vi "add_light-dark_j-t_measurements_to_queue.vi"(10 "Scan settings array":T3[](array[typedef]) {"J-t Illumination conditions" items=["Light only", "Dark only", "Light then dark", "Dark then light"]; "No. of scan rate steps" min=1.0 step=1.0; "Illumination conditions" items=["Light only", "Dark only", "Light then dark", "Dark then light", "Light then dark then light", "Dark then light then dark"]; "Only repeat for best pixel" items=["only for best pixel", "for best 2 pixels", "for best 3 pixels", "for best 4 pixels", "for best 5 pixels", "for best 6 pixels", "for best 7 pixels", "for all pixels"]; "No. of repeat scans" min=1.0 step=1.0; "Max power best pixel only" items=["only the best pixel", "the best 2 pixels", "the best 3 pixels", "the best 4 pixels", "the best 5 pixels", "the best 6 pixels", "the best 7 pixels", "all pixels"]; "J-t best pixel only" items=["only the best pixel", "the best 2 pixels", "the best 3 pixels", "the best 4 pixels", "the best 5 pixels", "the best 6 pixels", "the best 7 pixels", "all pixels"]; "Integration time" items=["Fast", "Normal", "High Accuracy"]; "Stabilisation mode" items=["V", "I"]; "Measurement delay (ms)" min=10.0}, 11 "Cell settings cluster":T2) -> (3 "Light/dark array":T1(array[cluster]))   [LabVIEW 2016]
uses:
  TypeDefs/scan_settings.ctl
  TypeDefs/Settings Boolean.ctl
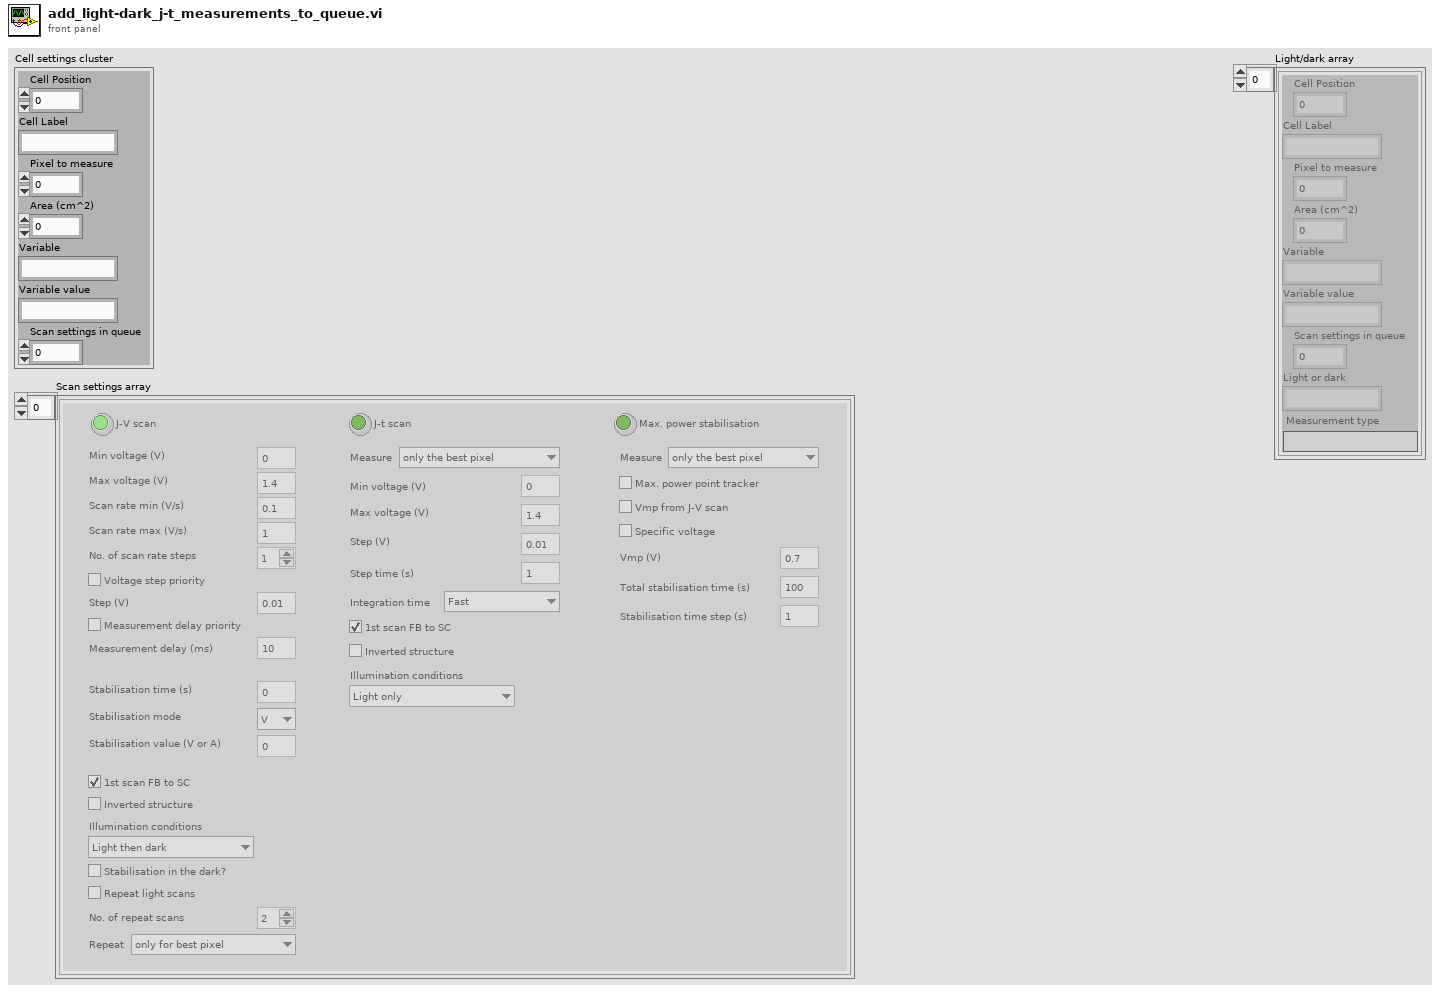
[diagram p1: front panel]
types:
  T1 = cluster{"Cell Position":i32, "Cell Label":string, "Pixel to measure":u16, "Area (cm^2)":dbl, "Variable":string, "Variable value":string, "Scan settings in queue":u16, "Light or dark":string, "Measurement type":string}[]
  T2 = cluster{"Cell Position":i32, "Cell Label":string, "Pixel to measure":u16, "Area (cm^2)":dbl, "Variable":string, "Variable value":string, "Scan settings in queue":u16}
  T3 = typedef "scan_settings.ctl" = cluster{"J-V scan":T4, "J-t scan":bool, "Min voltage (V)":dbl, "Max voltage (V)":dbl, "Step (V)":dbl, "Measurement delay (ms)":dbl, "1st scan FB-SC":bool, "Inverted structure":bool, "Stabilisation time (s)":dbl, "Stabilisation mode":u16, "Stabilisation value (V or A) ":dbl, "Step time (s)":dbl, "Integration time":u16, "Repeat light scans":bool, "Stabilisation in the dark?":bool, "J-t Min (V)":dbl, "J-t Max (V)":dbl, "J-t Step (V)":dbl, "Max. power stabilisation":bool, "J-t 1st scan FB-SC":bool, "J-t Inverted structure":bool, "Max power tracking":bool, "Vmp (V)":dbl, "Total stabilisation time (s)":dbl, "J-t best pixel only":u16, "Max power best pixel only":u16, "Vmp from J-V scan":bool, "No. of repeat scans":dbl, "Only repeat for best pixel":u16, "Stabilisation time step (s)":dbl, "Illumination conditions":u16, "Scan rate min (V/s)":dbl, "Scan rate max (V/s)":dbl, "No. of scan rate steps":dbl, "Scan rate voltage step priority":bool, "Scan rate measurement delay priority":bool, "J-t Illumination conditions":u16, "Max P stab. Specific voltage":bool}
  T4 = typedef "Settings Boolean.ctl" = bool
  T5 = cluster{"Cell Position":i32, "Cell Label":string, "Pixel to measure":u16, "Area (cm^2)":dbl, "Variable":string, "Variable value":string, "Scan settings in queue":u16, "Light or dark":string, "Measurement type":string}
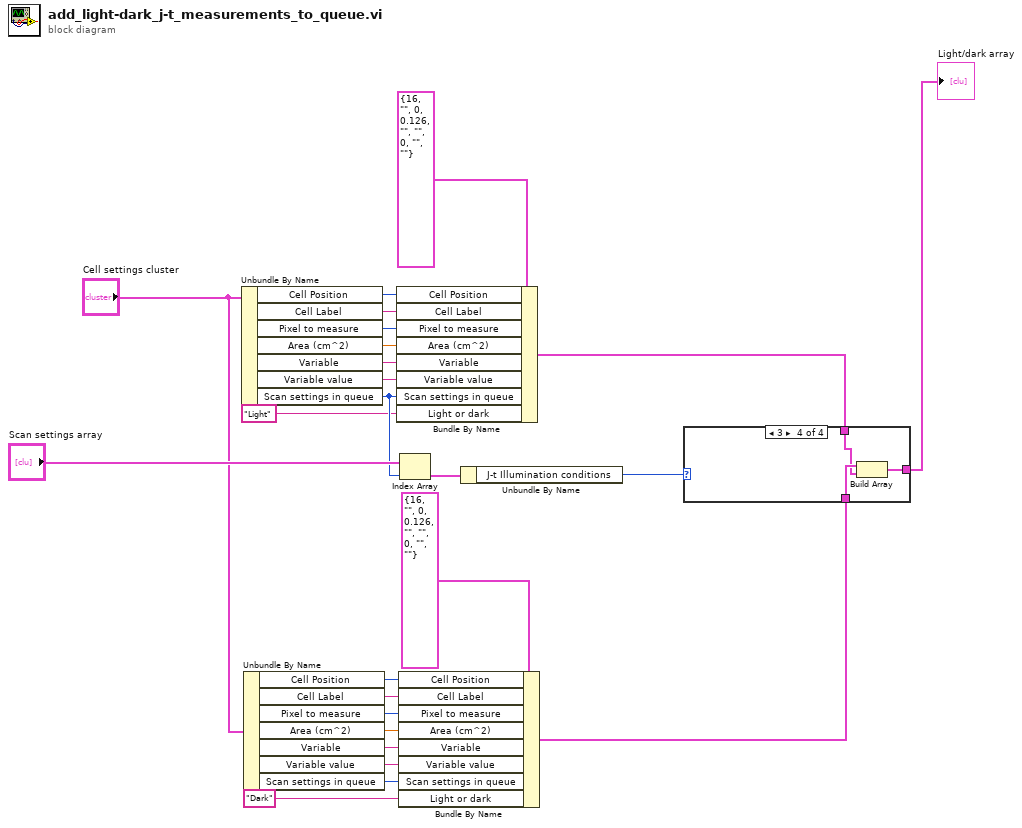
[diagram p0: block diagram]
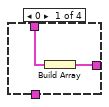
[diagram p2: hidden frame]
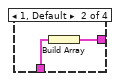
[diagram p3: hidden frame]
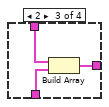
[diagram p4: hidden frame]
diagram:
  n1 = Unbundle By Name("Cell settings cluster") -> ("Cell Position"=w5:i32, "Cell Label"=w6:string, "Pixel to measure"=w7:u16, "Area (cm^2)"=w8:dbl, "Variable"=w9:string, "Variable value"=w10:string, "Scan settings in queue"=w23:u16)
  n2 = Unbundle By Name("Cell settings cluster") -> ("Cell Position"=w12:i32, "Cell Label"=w13:string, "Pixel to measure"=w14:u16, "Area (cm^2)"=w15:dbl, "Variable"=w16:string, "Variable value"=w17:string, "Scan settings in queue"=w18:u16)
  n3 = Bundle By Name(cluster=T5 {"Cell Position"=16, "Cell Label"="", "Pixel to measure"=0, "Area (cm^2)"=0.126, "Variable"="", "Variable value"="", "Scan settings in queue"=0, "Light or dark"="", "Measurement type"=""} ("System Cluster"), "Cell Position"=w5, "Cell Label"=w6, "Pixel to measure"=w7, "Area (cm^2)"=w8, "Variable"=w9, "Variable value"=w10, "Scan settings in queue"=w23, "Light or dark"="Light") -> (w3:T5)
  n4 = Bundle By Name(cluster=T5 {"Cell Position"=16, "Cell Label"="", "Pixel to measure"=0, "Area (cm^2)"=0.126, "Variable"="", "Variable value"="", "Scan settings in queue"=0, "Light or dark"="", "Measurement type"=""} ("System Cluster"), "Cell Position"=w12, "Cell Label"=w13, "Pixel to measure"=w14, "Area (cm^2)"=w15, "Variable"=w16, "Variable value"=w17, "Scan settings in queue"=w18, "Light or dark"="Dark") -> (w20:T5)
  n5 = Index Array(array="Scan settings array", index=w23) -> (element=w25:T3)
  n6 = Unbundle By Name(w25) -> ("J-t Illumination conditions"=w1:u16)
  n7 = case shown="3" w1 {
    tunnel: w3 -> [w27 _ w32 w33]
    tunnel: w20 -> [_ w29 w30 w35]
    tunnel: [w26 w28 w31 w34] -> w21
    frame 0 {
      n8 = Build Array(w27) -> (w26:T1)
    }
    frame 1, Default {
      n9 = Build Array(w29) -> (w28:T1)
    }
    frame 2 {
      n10 = Build Array(w32, w30) -> (w31:T1)
    }
    frame 3 {
      n11 = Build Array(w35, w33) -> (w34:T1)
    }
  }
  "Light/dark array" <- w21
